vi "Fetch Check-out Details.vi"(0 "File Data Manager in":refnum<class "File Data Manager.lvclass">, 5 "Rooms Manager GUID":string, 7 "Room No":string, 11 "error in (no error)":errorcluster) -> (4 "File Data Manager out":refnum<class "File Data Manager.lvclass">, 15 "error out":errorcluster)   [LabVIEW 2023, in "File Data Manager.lvlib" / "File Data Manager.lvclass"]
uses:
  File Data Manager.lvclass
  <vilib>/ActorFramework/Actor/Actor.lvclass/Actor.ctl
  File Data Manager.lvclass/File Data Manager.ctl
  Interfaces/Incoming Hotel Management Tool Model Interface Messages/Update Check-out Details Msg/Update Check-out Details Msg.lvclass/Update Check-out Details Msg.ctl
  <vilib>/ActorFramework/Message Enqueuer/Message Enqueuer.lvclass/Message Enqueuer.ctl
  <vilib>/ActorFramework/Message Enqueuer/Enqueue.vi
  Interfaces/Incoming Hotel Management Tool Model Interface Messages/Update Check-out Details Msg/Update Check-out Details Msg.lvclass
  <vilib>/ActorFramework/Message Priority Queue/Priority Enqueue.vi
  <vilib>/ActorFramework/Actor/Actor.lvclass
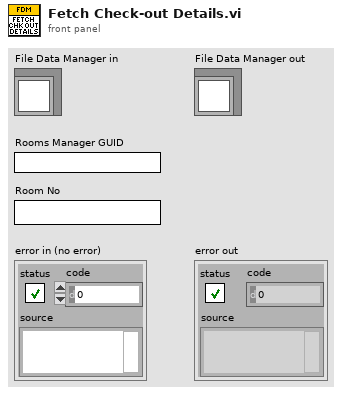
[diagram p1: front panel]
types:
  T1 = typedef "Central Data Manager.lvlib/Central Data Manager.lvclass/Room Size Details.ctl" = cluster{"Size":string, "Cost Per Day (Rs)":u32, "Occupancy Limit (Adult)":u32, "Occupancy Limit (Children)":u32}
  T2 = typedef "Central Data Manager.lvlib/Central Data Manager.lvclass/Room Details.ctl" = cluster{"Room No":string, "Room Size":string, "Room Occupancy Status":T3, "Guest Details":T4, "Occupancy Count (Adult)":u32, "Occupancy Count (Children)":u32, "Check-in Time":timestamp, "Check-out Time":timestamp}
  T3 = typedef "Central Data Manager.lvlib/Central Data Manager.lvclass/Room Occupancy Status.ctl" = enum16{"Not Occupied", "Occupied", "Under Maintainance", "Not Servicable"}
  T4 = typedef "Central Data Manager.lvlib/Central Data Manager.lvclass/Guest Details.ctl" = cluster{"Contact Number":string, "Primary Guest Name":string}
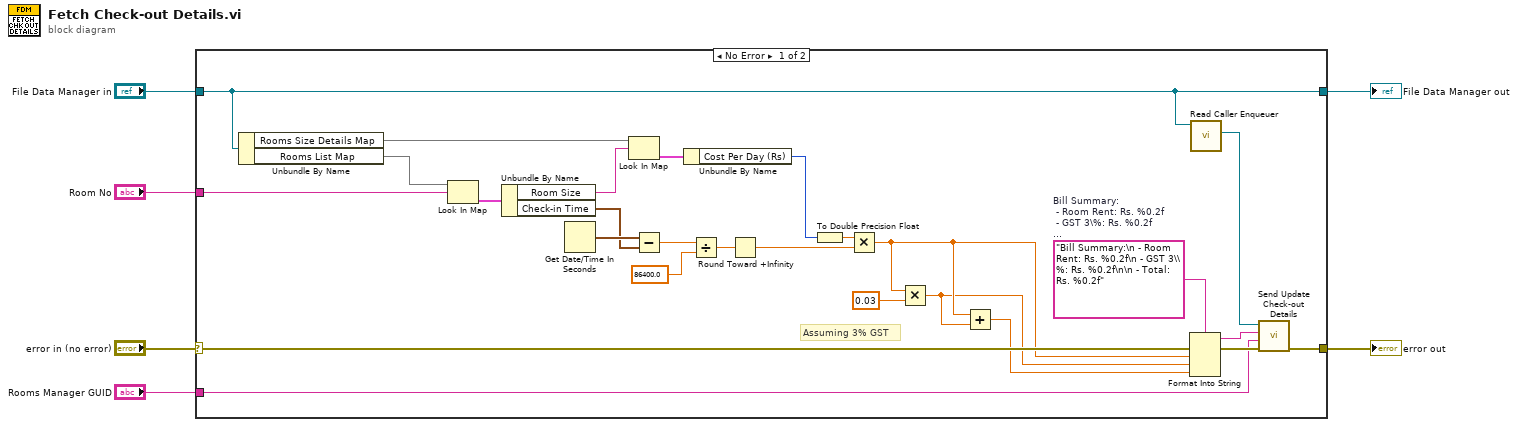
[diagram p0: block diagram]
diagram:
  n1 = case shown="No Error" "error in (no error)" {
    selector: "error in (no error)" -> [w27 w33]
    tunnel: [w26 w33] -> w5
    tunnel: "Rooms Manager GUID" -> [w11 _]
    tunnel: "File Data Manager in" -> [w25 w34]
    tunnel: "Room No" -> [w31 _]
    tunnel: [w25 w34] -> w1
    frame No Error {
      w12 = "Bill Summary:\n - Room Rent: Rs. %0.2f\n - GST 3\\%: Rs. %0.2f\n\n - Total: Rs. %0.2f"  # Bill Summary:  - Room Rent: Rs. %0.2f  - GST 3\%: Rs. %0.2f   - Total: Rs. %0.2f
      # "Assuming 3% GST"
      n2 = Unbundle By Name(w25) -> ("Rooms Size Details Map"=w29:map{string, T1}, "Rooms List Map"=w32:map{string, T2})
      n3 = Look In Map(map=w32, key=w31) -> (value=w30:T2)  [unwired: 1 in, 1 out]
      n4 = Unbundle By Name(w30) -> ("Room Size"=w28:string, "Check-in Time"=w21:timestamp)
      n5 = Get Date/Time In Seconds() -> (seconds since 1Jan1904=w22:timestamp)
      n6 = Look In Map(map=w29, key=w28) -> (value=w23:T1)  [unwired: 1 in, 1 out]
      n7 = Subtract(x=w22, y=w21) -> (x-y=w20:dbl)
      n8 = Unbundle By Name(w23) -> ("Cost Per Day (Rs)"=w17:u32)
      n9 = Divide(x=w20, y=86400.0) -> (x/y=w18:dbl)
      n10 = Round Toward +Infinity(x=w18) -> (ceil(x): smallest int >= x=w16:dbl)
      n11 = To Double Precision Float(number=w17) -> (double precision float=w15:dbl)
      n12 = Multiply(x=w15, y=w16) -> (x*y=w9:dbl)
      n13 = Multiply(x=w9, y=0.03) -> (x*y=w8:dbl)
      n14 = Add(x=w9, y=w8) -> (x+y=w7:dbl)
      n15 = Format Into String(format string=w12, error in=w27, w9, w8, w7) -> (resulting string=w13:string, error out=w14:errorcluster)  [unwired: 1 in]
      n16 = call <vilib>:"Read Caller Enqueuer.vi"("Actor"=w25) -> ("Caller Enqueuer"=w24:refnum<class "Message Enqueuer.lvclass">)  [unwired: 10 in]
      n17 = call "Send Update Check-out Details.vi"("error in (no error)"=w14, "Rooms Manager GUID"=w11, "Bill Summary"=w13, "Message Enqueuer"=w24) -> ("error out"=w26:errorcluster)  [unwired: 6 in, 1 out]
    }
    frame Error {
    }
  }
  "error out" <- w5
  "File Data Manager out" <- w1
